vi "RemoteControl.SendMessageFromProcess.vi"(8 "error in (no error)":errorcluster, 10 "Message":T1, 11 "RemoteControl":refnum<class "RemoteControl.lvclass">) -> (0 "error out":errorcluster, 3 "RemoteControl out":refnum<class "RemoteControl.lvclass">)   [LabVIEW 2019, in "RemoteControl.lvlib" / "RemoteControl.lvclass"]
doc: "---------------------------------------------------------------\nJKI State Machine Objects™\nhttp://jki.net/state-machine-objects/\nCopyright (C) 2005-2015, JKI <info@jki.net>\nALL RIGHTS RESERVEDJKI State Machine Objects (SMO) 1.0.0.4\nJKI - JKI\nCopyright (c) 2015, JKI"
uses:
  RemoteControl.lvclass
  Typedefs/Message--Cluster.ctl
  RemoteControl.lvclass/RemoteControl.ctl
  Typedefs/PublicEvents--RemoteControl.SendMessageFromProcess.ctl
panel:
  # "For instructions on how to use the JKI State Machine Objects, examples and video tutorials, visit:\nhttp://jki.net/state-machine-objects/\n\nJKI State Machine Objects™\nhttp://jki.net/state-machine-objects/\nCopyright (C) 2005-2015, JKI <info@jki.net>\nALL RIGHTS RESERVED"
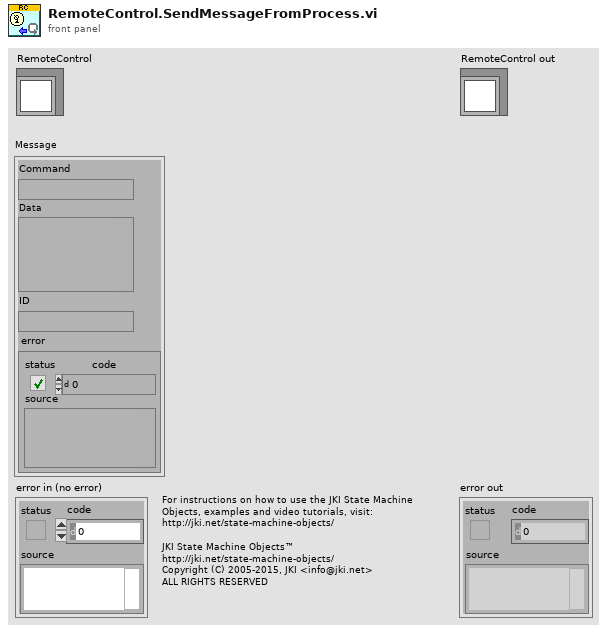
[diagram p1: front panel]
types:
  T1 = typedef "RemoteControl.lvlib/RemoteControl.lvclass/Message--Cluster.ctl" = cluster{"Command":string, "Data":variant, "ID":string, "error":errorcluster}
  T2 = typedef "RemoteControl.lvlib/RemoteControl.lvclass/PublicEvents--RemoteControl.SendMessageFromProcess.ctl" = cluster{"Message":T1}
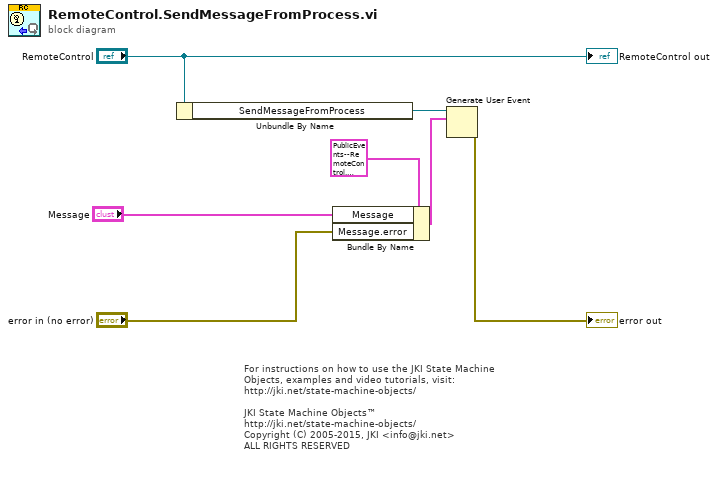
[diagram p0: block diagram]
diagram:
  # "For instructions on how to use the JKI State Machine Objects, examples and video tutorials, visit:\nhttp://jki.net/state-machine-objects/\n\nJKI State Machine Objects™\nhttp://jki.net/state-machine-objects/\nCopyright (C) 2005-2015, JKI <info@jki.net>\nALL RIGHTS RESERVED"
  n1 = Unbundle By Name("RemoteControl") -> ("SendMessageFromProcess"=w4:refnum<user-event>)
  n2 = Bundle By Name(cluster=T2 {"Message"={"Command"="", "Data"=variant(string ""), "ID"="", "error"={"status"=FALSE, "code"=0, "source"=""}}} ("SendMessageFromProcess"), "Message"="Message", "Message.error"="error in (no error)") -> (w2:T2)
  n3 = Generate User Event(user event=w4, event data cluster=w2) -> (error out=→"error out":errorcluster)  [unwired: 2 in, 1 out]
  "RemoteControl out" <- "RemoteControl"
